vi "RTP_RTSP - PLAY - METHOD.vi"(0 "RTSP Session":T1, 9 "timeout ms (1000)":i32=1000, 11 "error in (no error)":errorcluster) -> (4 "RTSP Session 2":T1, 15 "error out":errorcluster)   [LabVIEW 2014]
uses:
  RTSP Session.ctl
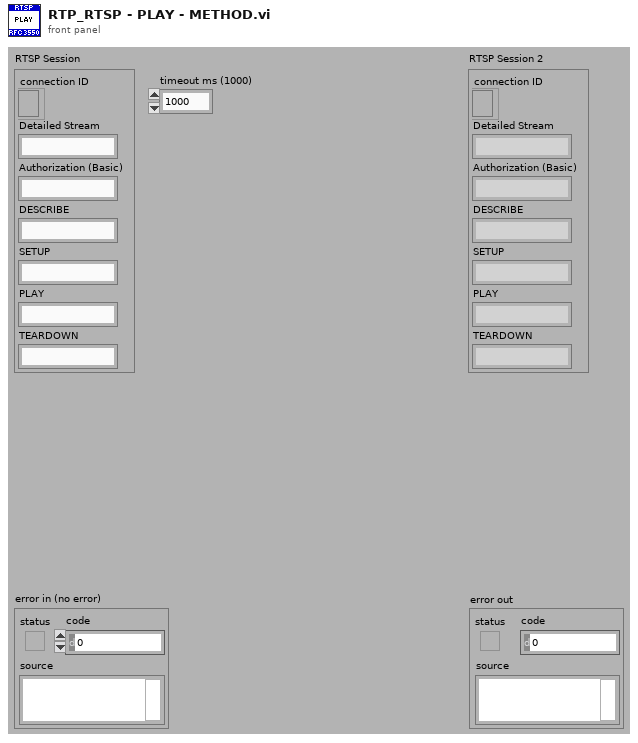
[diagram p1: front panel]
types:
  T1 = typedef "RTSP Session.ctl" = cluster{"connection ID":refnum<k5>, "Authorization (Basic)":string, "Detailed Stream":string, "DESCRIBE":string, "SETUP":string, "PLAY":string, "TEARDOWN":string}
  T2 = enum16{"Standard", "Buffered", "CRLF", "Immediate"}
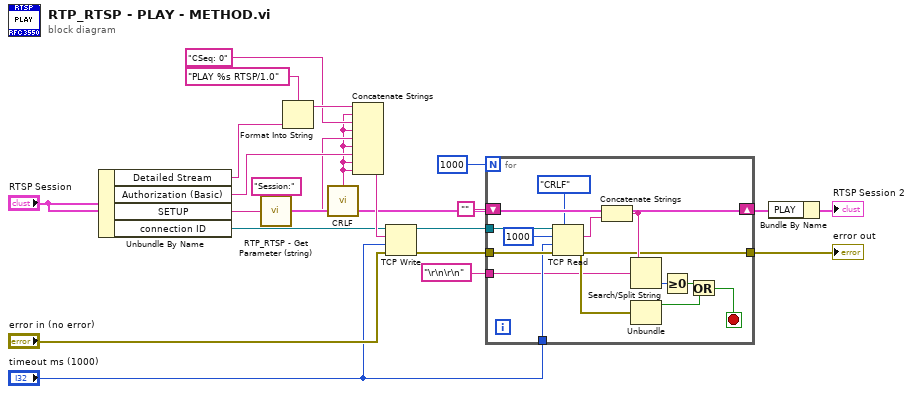
[diagram p0: block diagram]
diagram:
  n1 = Unbundle By Name("RTSP Session") -> ("Detailed Stream"=w9:string, "Authorization (Basic)"=w8:string, "SETUP"=w6:string, "connection ID"=w11:refnum<k5>)
  n2 = call "RTP_RTSP - Get Parameter (string).vi"("Name"="Session:" ("search string/char (-)"), "Data"=w6) -> ("Parameter"=w2:string)  [unwired: 13 in]
  n3 = Format Into String(format string="PLAY %s RTSP/1.0", w9) -> (resulting string=w20:string)  [unwired: 2 in, 1 out]
  n4 = call "CRLF.vi"() -> ("CRLF"=w1:string)
  n5 = Concatenate Strings(w20, w1, "CSeq: 0" ("string"), w1, w2, w1, w8, w1, w1) -> (w19:string)
  n6 = TCP Write(connection ID=w11, data in=w19, error in (no error)="error in (no error)", 9:"timeout ms (1000)") -> (connection ID out=w15:refnum<k5>, error out=w14:errorcluster)  [unwired: 1 out]
  n7 = for {
    N: 1000 -> [_]
    tunnel: w14 -> [w36]
    tunnel: w15 -> [w35]
    tunnel: [w27] -> w12
    shift-right: [w29] -> w3
    shift-left: "" -> [w33]
    tunnel: "timeout ms (1000)" -> [w30]
    tunnel: "\r\n\r\n" ("search string/char (-)") -> [w26]
    stop <- w23 stop-if-true
    n8 = TCP Read(connection ID=w35, bytes to read=1000, error in (no error)=w36, 7:T2."CRLF" ("mode (standard)"), 9:w30) -> (data out=w32:string, error out=w27:errorcluster)  [unwired: 1 out]
    n9 = Concatenate Strings(w33, w32) -> (w29:string)
    n10 = Search/Split String(string=w29, search string/char (-)=w26) -> (offset of match=w28:i32)  [unwired: 1 in, 2 out]
    n11 = Unbundle(w27) -> ("status"=w24:bool)  [unwired: 2 out]
    n12 = Greater Or Equal To 0?(x=w28) -> (x >= 0?=w25:bool)
    n13 = Or(x=w25, y=w24) -> (x .or. y?=w23:bool)
  }
  "error out" <- w12
  n14 = Bundle By Name(cluster="RTSP Session", "PLAY"=w3) -> (→"RTSP Session 2":T1)
